vi "DOF Index Write.vi"(4 "error in (no error)":errorcluster, 5 "Value":i32, 6 "Container State":T5, 7 "Display State In":T1) -> (0 "error out":errorcluster, 3 "Display State Out":T1)   [LabVIEW 2013, in "Limits X.xctl"]
uses:
  Limits X.xctl
  <vilib>/_xctls/Container State.ctl
  Limits State.ctl
  lib/Data Access Objects/Limits/DofTypes.ctl
  lib/Limits/Limite State.ctl
  lib/Apps/Yes No Button.ctl
  <vilib>/_xctls/XControlSupport.lvlib
panel:
  # "Replace the Value Control below with a Control of desired type.\nDo not remove this Control or the others from the connector pane.\nDo not change the connector pane pattern.\nThe Value control should always be the third terminal from top on the input side in the connector pane."
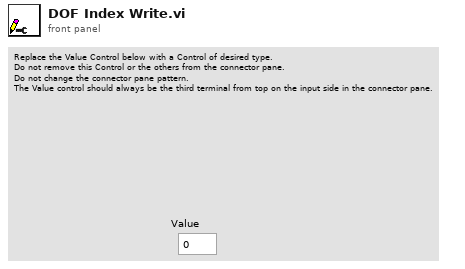
[diagram p1: front panel]
types:
  T1 = typedef "Limits X.xctl/Limits State.ctl" = cluster{"DofType":T2, "Limit State":T3, "DOF Index":i32, "System Fault ":T4, "Has Lower":T4}
  T2 = typedef "DofTypes.ctl" = enum16{"Cartesian Displacements", "Cartesian Forces & Moments", "Actuator Displacements", "Actuator Forces", "Cartesian Increments", "Actuator Increments"}
  T3 = typedef "Limite State.ctl" = enum16{"Good", "Lower Bound Fault", "Upper Bound Fault"}
  T4 = typedef "Yes No Button.ctl" = bool
  T5 = typedef "XControlSupport.lvlib/Container State.ctl" = cluster{"Indicator?":bool, "Run Mode?":bool, " Refnum":refnum<vi>}
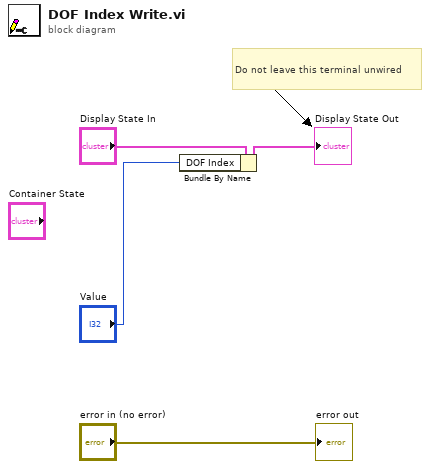
[diagram p0: block diagram]
diagram:
  # "Do not leave this terminal unwired"
  n1 = Bundle By Name(cluster="Display State In", "DOF Index"="Value") -> (→"Display State Out":T1)
  "error out" <- "error in (no error)"
